vi "Configure Device.vi"(8 "error in":errorcluster, 11 "PPT in":refnum<class "PPT.lvclass">) -> (0 "error out":errorcluster, 3 "PPT out":refnum<class "PPT.lvclass">)   [LabVIEW 2014, in "PPT.lvclass"]
uses:
  PPT.lvclass
  Reusable/Session APIs/Text Communication/Text Device Session.lvclass
  PPT.lvclass/PPT.ctl
  Configurable Device/Configurable Device.lvclass/Configurable Device.ctl
  Reusable/Session APIs/Text Communication/Text Device Session.lvclass/Text Device Session.ctl
  Reusable/Session APIs/File Access/Config Data/Config Data.lvclass/Config Data.ctl
  Accessors/Read ID.vi
  Accessors/Read hSession.vi
  Configurable Device/Read Handle.vi
  Reusable/Session APIs/Text Communication/Read hSysLog.vi
  Reusable/Session APIs/File Access/Config Data/Accessors/Read Ref.vi
  Accessors/Write ID.vi
  <vilib>/Utility/config.llb/Read Key (I32).vi
  <vilib>/Utility/config.llb/Read Key (String).vi
  <userlib>/_Session Fwk/Session - Root.lvclass
  Reusable/Session APIs/File Access/Config Data/Config Data.lvclass
  <vilib>/Utility/config.llb/NI_LVConfig.lvlib
  Reusable/Session Log/System Log.lvclass
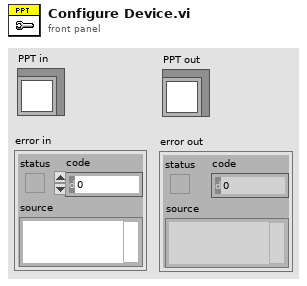
[diagram p1: front panel]
types:
  T1 = typedef "Session - Root.lvclass/Session Handle.ctl" = refnum<data-value>
  T2 = typedef "Config Data.lvclass/Config Session.ctl" = refnum<data-value>
  T3 = typedef "NI_LVConfig.lvlib/Config Data RefNum.ctl" = refnum<k1>
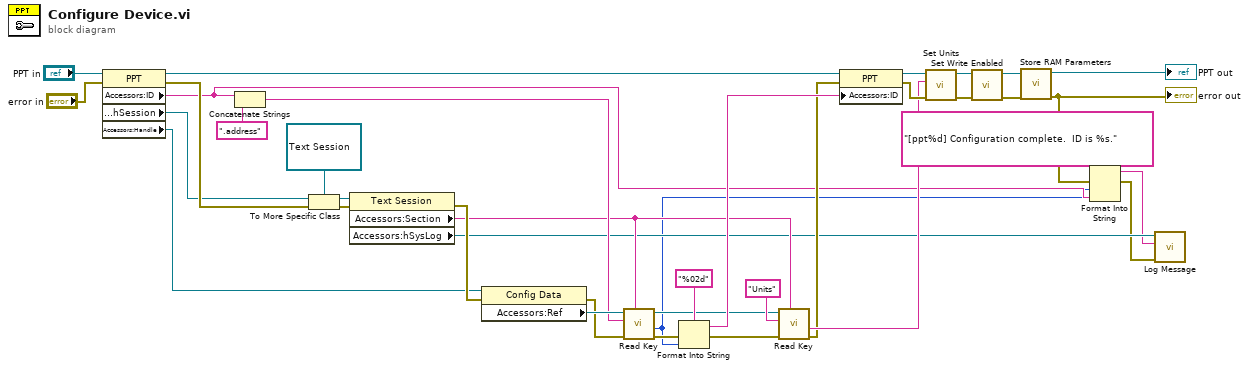
[diagram p0: block diagram]
diagram:
  n1 = property class="PPT"(reference="PPT in", error in="error in") -> (reference out=w29:refnum<class "PPT.lvclass">, error out=w15:errorcluster, "Accessors:ID"=w2:string, "Accessors:hSession"=w14:T1, "Accessors:Handle"=w17:T2)
  n2 = Concatenate Strings(w2, ".address" ("string")) -> (w31:string)
  n3 = To More Specific Class(target class=refnum<data-value> refnum ("hSession"), reference=w14, error in=w15) -> (specific class reference=w35:refnum<data-value>, error out=w34:errorcluster)
  n4 = property class="Text Session"(reference=w35, error in=w34) -> (error out=w27:errorcluster, "Accessors:Section"=w13:string, "Accessors:hSysLog"=w7:T1)  [unwired: 1 out]
  n5 = property class="Config Data"(reference=w17, error in=w27) -> (error out=w26:errorcluster, "Accessors:Ref"=w33:T3)  [unwired: 1 out]
  n6 = call-poly <vilib>:"Read Key.vi"("section"=w13, "error in (no error)"=w26, "key"=w31, "refnum"=w33) -> ("error out"=w25:errorcluster, "value"=w1:i32, "refnum out"=w10:T3)  [unwired: 4 in, 1 out]
  n7 = Format Into String(format string="%02d", error in=w25, w1) -> (resulting string=w28:string, error out=w11:errorcluster)  [unwired: 1 in]
  n8 = call-poly <vilib>:"Read Key.vi"("section"=w13, "error in (no error)"=w11, "key"="Units", "refnum"=w10) -> ("error out"=w8:errorcluster, "value"=w9:string)  [unwired: 4 in, 2 out]
  n9 = property class="PPT"(reference=w29, error in=w8, "Accessors:ID"=w28) -> (reference out=w24:refnum<class "PPT.lvclass">, error out=w23:errorcluster)
  n10 = call "Set Units.vi"("error in"=w23, "Units"=w9, "PPT in"=w24) -> ("error out"=w21:errorcluster, "PPT out"=w22:refnum<class "PPT.lvclass">)  [unwired: 7 in]
  n11 = call "Set Write Enabled.vi"("error in"=w21, "PPT in"=w22) -> ("error out"=w19:errorcluster, "PPT out"=w20:refnum<class "PPT.lvclass">)  [unwired: 8 in]
  n12 = call "Store RAM Parameters.vi"("error in"=w19, "PPT in"=w20) -> ("error out"=w3:errorcluster, "PPT out"=→"PPT out":refnum<class "PPT.lvclass">)  [unwired: 8 in]
  "error out" <- w3
  n13 = Format Into String(format string="[ppt%d] Configuration complete.  ID is %s.", error in=w3, w1, w2) -> (resulting string=w5:string, error out=w4:errorcluster)  [unwired: 1 in]
  n14 = call "Log Message.vi"("error in"=w4, "MSG In"=w5, "session in"=w7) -> ()  [unwired: 7 in, 2 out]
